vi "LVClass_ClosedLoopSecurity_Ctor.vi"(0 "ClosedLoopSecurity const)":refnum<class "ClosedLoopSecurity.lvclass">, 5 "ClosedLoopSecurityParams":T1, 11 "error in (no error)":errorcluster) -> (4 "ClosedLoopSecurity (new)":refnum<class "ClosedLoopSecurity.lvclass">, 15 "error out":errorcluster)   [LabVIEW 2020, in "ClosedLoopSecurity.lvclass"]
doc: "Manual construction.\n\n<B>security_paramsIn</B> : Constant Pointer to Closed Loop security params object.\n<B>security_paramsOut</B> : Constant Pointer to Closed Loop security params object.\n<B>max_saturated_act_count</B> : Maximum tolerated count of saturated actuators\n<B>max_camera_fill_pct</B> : Maximum tolerated saturation percentage on camera signal\n<B>max_pupil_size_variation</B> : Maximum tolerated variation of the pupil size, relatively to the command\n matrix pupil size\n<B>max_dwf_pv</B> : Maximum tolerated delta wavefront peak-to-valley"
uses:
  ClosedLoopSecurity.lvclass
  Controls/ClosedLoopSecurityParameters.ctl
  Controls/Handle creation.ctl
  ClosedLoopSecurity.lvclass/ClosedLoopSecurity.ctl
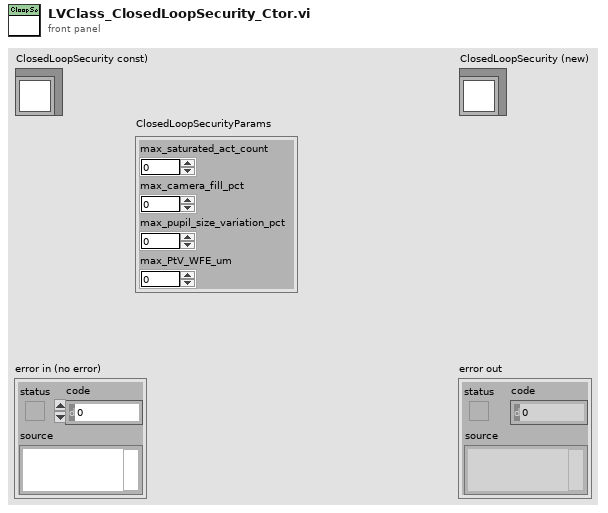
[diagram p1: front panel]
types:
  T1 = typedef "ClosedLoopSecurityParameters.ctl" = cluster{"max_saturated_act_count":i32, "max_camera_fill_pct":i32, "max_pupil_size_variation_pct":i32, "max_PtV_WFE_um":sgl}
  T2 = typedef "Handle creation.ctl" = enum16{"By ctor", "By write function"}
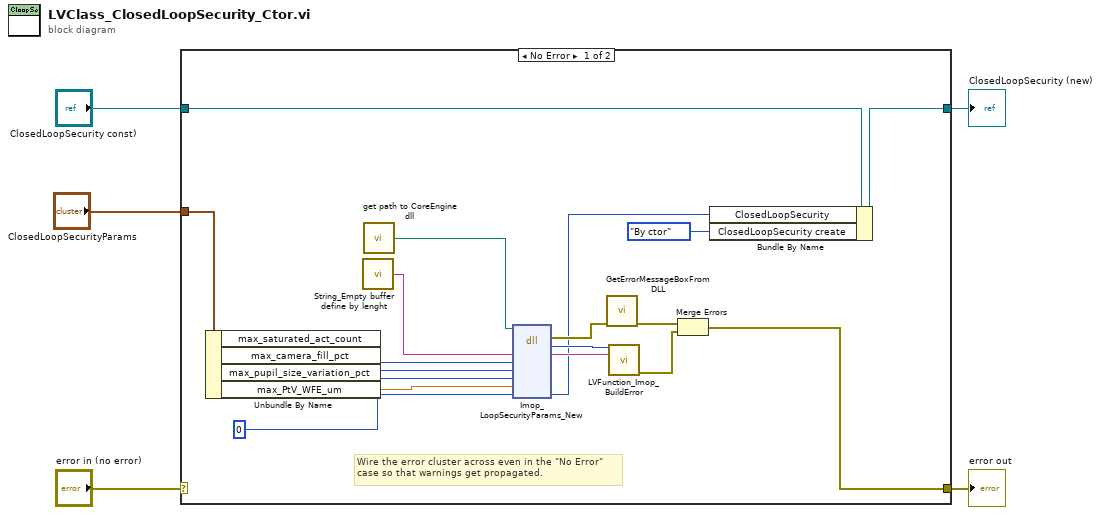
[diagram p0: block diagram]
diagram:
  n1 = case shown="No Error" "error in (no error)" {
    selector: "error in (no error)" -> [_ w25]
    tunnel: [w11 w25] -> w4
    tunnel: [w12 w24] -> w2
    tunnel: "ClosedLoopSecurity const)" -> [w13 w24]
    tunnel: "ClosedLoopSecurityParams" -> [w10 _]
    frame No Error {
      # "Wire the error cluster across even in the \"No Error\"\ncase so that warnings get propagated."
      n2 = Unbundle By Name(w10) -> ("max_saturated_act_count"=w9:i32, "max_camera_fill_pct"=w8:i32, "max_pupil_size_variation_pct"=w7:i32, "max_PtV_WFE_um"=w6:sgl)
      n3 = call "String_Empty buffer define by lenght.vi"() -> ("Empty buffer"=w23:string)  [unwired: 1 in]
      n4 = call "get path to CoreEngine dll.vi"() -> ("path to wavekit library"=w14:path)  [unwired: 14 in, 1 out]
      n5 = dll-call lib="D:/soft/HASO_v3/SVN_trunk/ImOpCoreEngine4_LV2011/DLLs/c_interface_vc100.dll" fn="Imop_LoopSecurityParams_New"(path in=w14, "message"=w23, "max_saturated_act_count"=w9, "max_camera_fill_pct"=w8, "max_pupil_size_variation"=w7, "max_loop_gain"=w6, "security_params"=0 ("Pupil")) -> (error out=w20:errorcluster, "return type"=w21:i32, "message"=w22:string, "security_params"=w18:i64)  [unwired: 6 in, 1 out]
      n6 = call "GetErrorMessageBoxFromDLL.vi"("error IN"=w20) -> ("error OUT"=w16:errorcluster)  [unwired: 10 in]
      n7 = call "LVFunction_Imop_BuildError.vi"("code"=w21, "String to Prepend to source (\"\")"=w22) -> ("error out"=w15:errorcluster)  [unwired: 13 in]
      n8 = Merge Errors(w16, w15) -> (w11:errorcluster)
      n9 = Bundle By Name(cluster=w13, "ClosedLoopSecurity"=w18, "ClosedLoopSecurity create"=Handle_creation."By ctor" ("Pupil ptr create")) -> (w12:refnum<class "ClosedLoopSecurity.lvclass">)
    }
    frame Error {
    }
  }
  "error out" <- w4
  "ClosedLoopSecurity (new)" <- w2
